vi "picoscope5000a acquire.vi"(0 "handle in":i16, 1 "Ranges":u16[](array[numeric])=[6, 6], 5 "enabled array":i16[](array[numeric]), 7 "Max ADC value":i16, 9 "Device Info":T2, 11 "error in (no error)":errorcluster, 12 "Rapid Block Acquisition Settings":T3) -> (4 "Properties Panel":T1 {"Max Total Capture Time Available (sec)" format="%.3p"; "Sample Frequency" format="%.3p"; "Sample Rate" format="%.3p"; "Max Samples Available" format="%.3p"; "Total Capture Time (sec)" format="%.3p"}, 6 "handle out":i16, 8 "Waveform Data":waveform(dbl)[](graph), 10 "Num samples":u32, 15 "error out":errorcluster)   [LabVIEW 2020]
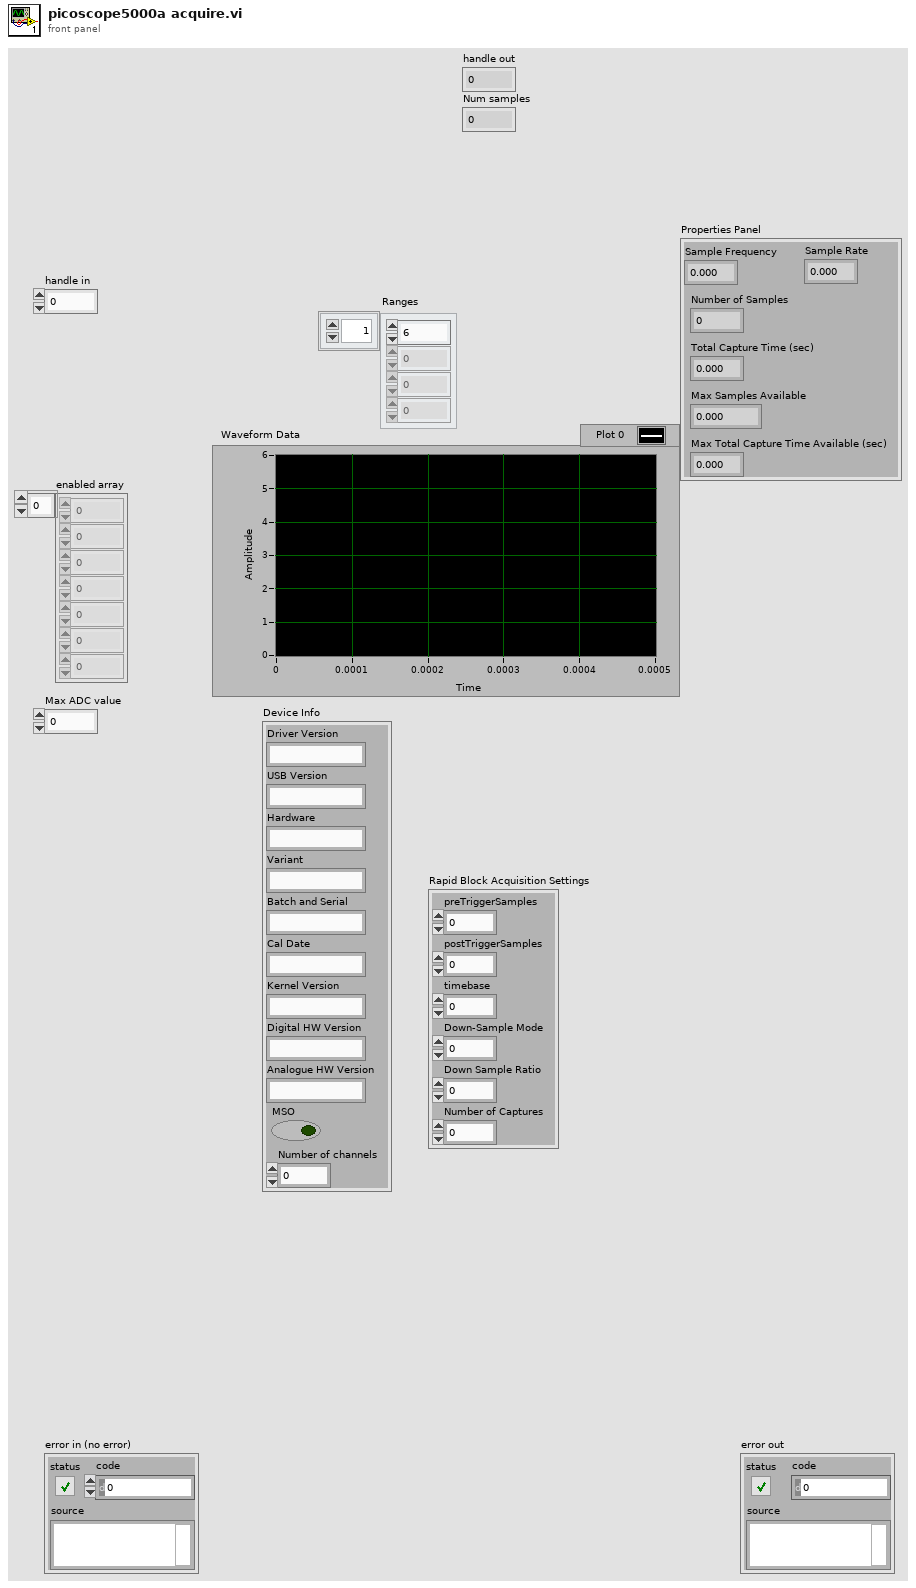
[diagram p1: front panel]
types:
  T1 = cluster{"Sample Frequency":sgl, "Sample Rate":sgl, "Max Samples Available":i32, "Number of Samples":u32, "Total Capture Time (sec) ":sgl, "Max Total Capture Time Available (sec)":sgl}
  T2 = cluster{"Driver Version":string, "USB Version":string, "Hardware":string, "Variant":string, "Batch and Serial":string, "Cal Date":string, "Kernel Version":string, "Digital HW Version":string, "Analogue HW Version":string, "MSO":bool, "Number of channels":i16}
  T3 = cluster{"preTriggerSamples":u32, "postTriggerSamples":u32, "timebase":u32, "Down-Sample Mode":i32, "Down Sample Ratio":u32, "Number of Captures":u32}
  T4 = cluster{"preTriggerSamples":u32, "postTriggerSamples":u32, "timebase":u32, "Down-Sample Mode":i32, "Down Sample Ratio":u32}
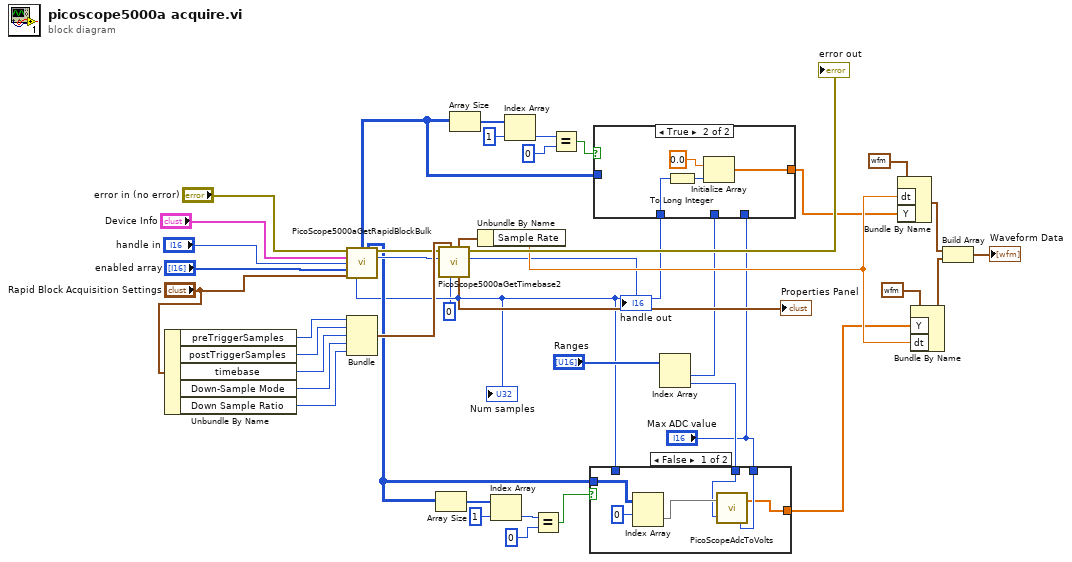
[diagram p0: block diagram]
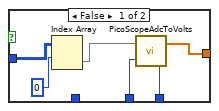
[diagram p2: hidden frame]
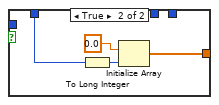
[diagram p3: hidden frame]
diagram:
  n1 = Unbundle By Name("Rapid Block Acquisition Settings") -> ("preTriggerSamples"=w37:u32, "postTriggerSamples"=w38:u32, "timebase"=w39:u32, "Down-Sample Mode"=w40:i32, "Down Sample Ratio"=w41:u32)
  n2 = call "PicoScope5000aGetRapidBlockBulk.vi"("error in"="error in (no error)", "Device Info"="Device Info", "handle in"="handle in", "enabled array"="enabled array", "Rapid Block Acquisition Settings"="Rapid Block Acquisition Settings") -> ("Channel A Buffer"=w3:i16[][], "Channel B Buffer"=w15:i16[][], "error out"=w31:errorcluster, "handle out"=w33:i16, "Num samples"=w5:u32)  [unwired: 2 in, 4 out]
  "Num samples" <- w5
  n3 = Bundle("preTriggerSamples"=w37, "postTriggerSamples"=w38, "timebase"=w39, "Down-Sample Mode"=w40, "Down Sample Ratio"=w41) -> (w36:T4)  [unwired: 1 in]
  n4 = Array Size(array=w15) -> (size(s)=w23:i32[])
  n5 = call "PicoScope5000aGetTimebase2.vi"("Number of Samples"=w5, "Memory Segment"=u32 0, "Acquisition Settings"=w36, "handle in"=w33, "error in (no error)"=w31) -> ("handle out"=→"handle out":i16, "error out"=→"error out":errorcluster, "Properties Panel"=w13:T1)  [unwired: 4 in]
  "Properties Panel" <- w13
  n6 = Array Size(array=w3) -> (size(s)=w8:i32[])
  n7 = Unbundle By Name(w13) -> ("Sample Rate"=w21:sgl)
  n8 = Index Array(array=w23, index=1) -> (element=w19:i32)
  n9 = Index Array(array=w8, index=1) -> (element=w11:i32)
  n10 = Equal?(x=w19, y=0) -> (x = y?=w18:bool)
  n11 = Equal?(x=w11, y=0) -> (x = y?=w10:bool)
  n12 = Index Array(array="Ranges") -> (element #1=w7:u16, element #2=w16:u16)  [unwired: 2 in]
  n13 = case shown="False" w18 {
    tunnel: [w44 w51] -> w17
    tunnel: "Max ADC value" -> [w47 _]
    tunnel: w16 -> [w46 _]
    tunnel: w15 -> [w45 _]
    tunnel: w5 -> [_ w49]
    frame False {
      n14 = Index Array(array=w45, index (row)=0) -> (element=w48:i16[])  [unwired: 1 in]
      n15 = call "PicoScopeAdcToVolts.vi"("Max_adc"=w47, "Range Index"=w46, "Data"=w48) -> ("Data (Volts)"=w44:dbl[])
    }
    frame True {
      n16 = To Long Integer(number=w49) -> (32bit integer=w50:i32)
      n17 = Initialize Array(0.0 ("element"), w50) -> (w51:dbl[])
    }
  }
  n18 = case shown="True" w10 {
    tunnel: [w56 w61] -> w4
    tunnel: w3 -> [w57 _]
    tunnel: w5 -> [_ w59]
    tunnel: w7 -> [w55 _]
    tunnel: "Max ADC value" -> [w54 _]
    frame False {
      n19 = Index Array(array=w57, index (row)=0) -> (element=w58:i16[])  [unwired: 1 in]
      n20 = call "PicoScopeAdcToVolts.vi"("Max_adc"=w54, "Range Index"=w55, "Data"=w58) -> ("Data (Volts)"=w56:dbl[])
    }
    frame True {
      n21 = To Long Integer(number=w59) -> (32bit integer=w60:i32)
      n22 = Initialize Array(0.0 ("element"), w60) -> (w61:dbl[])
    }
  }
  n23 = Bundle By Name(cluster=waveform(dbl) {"t0"=timestamp(0 s since 1904-01-01), "dt"=1.0, "Y"=[]} ("Waveform Graph"), "dt"=w21, "Y"=w4) -> (w28:waveform(dbl))
  n24 = Bundle By Name(cluster=waveform(dbl) {"t0"=timestamp(0 s since 1904-01-01), "dt"=1.0, "Y"=[]} ("Waveform Graph"), "Y"=w17, "dt"=w21) -> (w27:waveform(dbl))
  n25 = Build Array(w28, w27) -> (→"Waveform Data":waveform(dbl)[])
